vi "Find Instrument Addon Custom Device.vi"(8 "error in":errorcluster, 11 "target in":refnum<k24>) -> (0 "error out":errorcluster, 1 "NodeID":u64, 3 "target out":refnum<k24>)   [LabVIEW 2023]
uses:
  NationalInstruments.VeriStand.SystemDefinitionAPI
  Addon/Addon Shared/SubVIs/Constants.vi
  Addon/Addon Shared/Instrument Addon Shared.lvlib
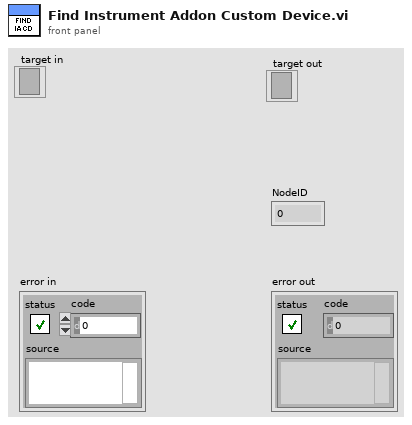
[diagram p1: front panel]
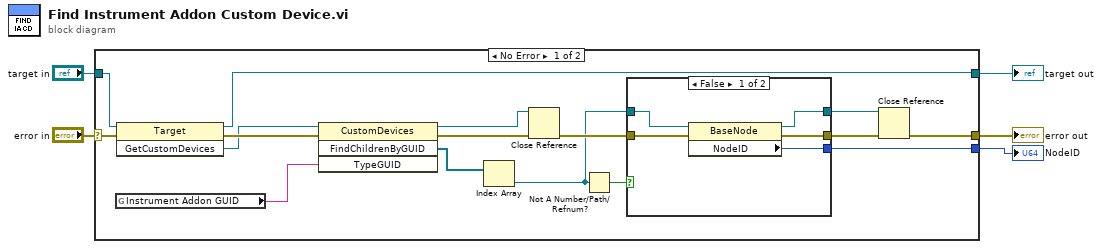
[diagram p0: block diagram]
diagram:
  n1 = case shown="No Error" "error in" {
    selector: "error in" -> [w21 w30]
    tunnel: [w10 w30] -> w5
    tunnel: "target in" -> [w20 w29]
    tunnel: [w14 w29] -> w2
    tunnel: [w12 _] -> w1
    frame No Error {
      n2 = global read "Constants.vi" "Instrument Addon GUID"() -> (w6:string)
      n3 = invoke class="Target" method="GetCustomDevices"(reference=w20, error in=w21) -> (reference out=w14:refnum<k24>, error out=w19:errorcluster, "GetCustomDevices"=w18:refnum<k24>)  [unwired: 1 in]
      n4 = invoke class="CustomDevices" method="FindChildrenByGUID"(reference=w18, error in=w19, "TypeGUID"=w6) -> (reference out=w17:refnum<k24>, error out=w16:errorcluster, "FindChildrenByGUID"=w8:refnum<k24>[])  [unwired: 1 in, 1 out]
      n5 = Index Array(array=w8) -> (element=w7:refnum<k24>)  [unwired: 1 in]
      n6 = Close Reference(reference=w17, error in (no error)=w16) -> (error out=w15:errorcluster)
      n7 = Not A Number/Path/Refnum?(number/path/refnum=w7) -> (NaN/Path/Refnum?=w13:bool)
      n8 = case shown="False" w13 {
        tunnel: [w22 w28] -> w9
        tunnel: w15 -> [w24 w28]
        tunnel: w7 -> [w26 w27]
        tunnel: [w25 _] -> w12
        tunnel: [w23 w27] -> w11
        frame False {
          n9 = property class="BaseNode"(reference=w26, error in=w24) -> (reference out=w23:refnum<k24>, error out=w22:errorcluster, "NodeID"=w25:u64)
        }
        frame True {
        }
      }
      n10 = Close Reference(reference=w11, error in (no error)=w9) -> (error out=w10:errorcluster)
    }
    frame Error {
    }
  }
  "target out" <- w2
  "error out" <- w5
  "NodeID" <- w1
